vi "TaskPool_get.vi"(8 "taskType":string, 10 "taskArr in":refnum<k21>[](array[refnum])) -> (1 "isNull":bool, 2 "taskhandle":refnum<k21>, 3 "taskArr out":refnum<k21>[](array[refnum]))   [LabVIEW 2016]
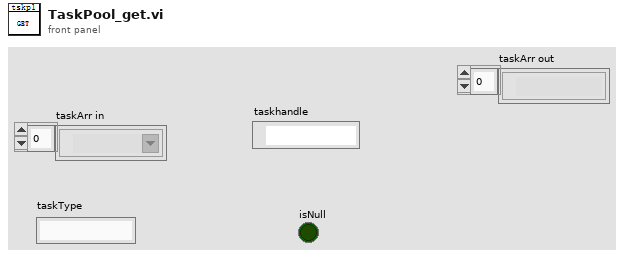
[diagram p1: front panel]
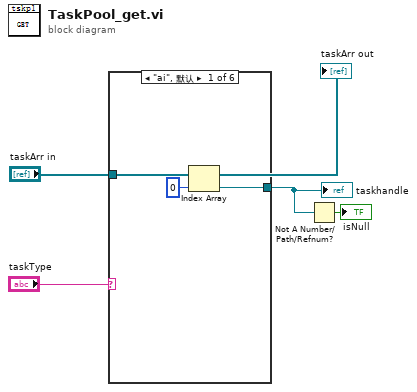
[diagram p0: block diagram]
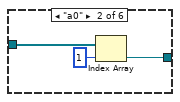
[diagram p2: hidden frame]
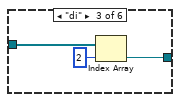
[diagram p3: hidden frame]
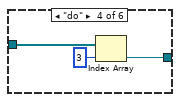
[diagram p4: hidden frame]
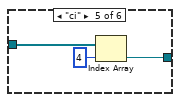
[diagram p5: hidden frame]
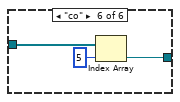
[diagram p6: hidden frame]
diagram:
  n1 = case shown="\"ai\", 默认" "taskType" {
    tunnel: "taskArr in" -> [w7 w10 w13 w16 w19 w22]
    tunnel: [w6 w9 w12 w15 w18 w21] -> w1
    frame "ai", Default {
      n2 = Index Array(array=w7, index=0 ("索引")) -> (element=w6:refnum<k21>)
    }
    frame "a0" {
      n3 = Index Array(array=w10, index=1 ("索引")) -> (element=w9:refnum<k21>)
    }
    frame "di" {
      n4 = Index Array(array=w13, index=2 ("索引")) -> (element=w12:refnum<k21>)
    }
    frame "do" {
      n5 = Index Array(array=w16, index=3 ("索引")) -> (element=w15:refnum<k21>)
    }
    frame "ci" {
      n6 = Index Array(array=w19, index=4 ("索引")) -> (element=w18:refnum<k21>)
    }
    frame "co" {
      n7 = Index Array(array=w22, index=5 ("索引")) -> (element=w21:refnum<k21>)
    }
  }
  "taskhandle" <- w1
  n8 = Not A Number/Path/Refnum?(number/path/refnum=w1) -> (NaN/Path/Refnum?=→"isNull":bool)
  "taskArr out" <- "taskArr in"
